vi "workspace.add_to_payload.vi"(8 "error in":errorcluster, 10 "JSON payload in":string, 11 "Nominal Client in":refnum<class "Nominal Client.lvclass">) -> (0 "error out":errorcluster, 1 "JSON payload out":string, 3 "Nominal Client out":refnum<class "Nominal Client.lvclass">)   [LabVIEW 2020, in "Nominal Client.lvclass"]
uses:
  Nominal Client.lvclass
  Nominal Client.lvclass/Nominal Client.ctl
  nominal types/workspace/workspace.lvclass/workspace.ctl
  88650e10-de3e-481c-85db-71cb0fdf4485.vi
  nominal types/workspace/rid.get.vi
  <vilib>/JDP Science/JSONtext/Variant to JSON Text.vi
  <vilib>/JDP Science/JSONtext/Get all Object Items.vi
  <vilib>/JDP Science/JSONtext/Set Multiple Object Items.vi
  <vilib>/JDP Science/JSONtext/LVClass Serializer/JSONtext LVClass Serializer.lvclass
  <vilib>/JDP Science/JSONtext/JSONtext.lvlib
  nominal types/workspace/workspace.lvclass
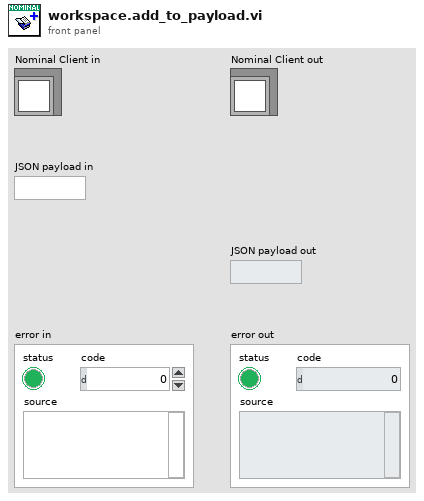
[diagram p1: front panel]
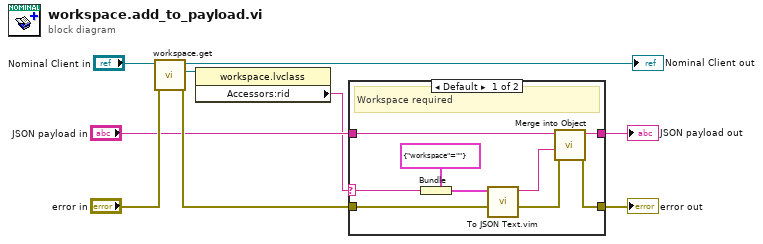
[diagram p0: block diagram]
diagram:
  n1 = call "workspace.get.vi"("error in"="error in", "Nominal Client in"="Nominal Client in") -> ("error out"=w6:errorcluster, "workspace"=w2:refnum<class "workspace.lvclass">, "Nominal Client out"=→"Nominal Client out":refnum<class "Nominal Client.lvclass">)  [unwired: 7 in]
  n2 = property class="workspace.lvclass"(reference=w2) -> ("Accessors:rid"=w1:string)  [unwired: 1 in, 2 out]
  n3 = case shown="Default" w1 {
    selector: w1 -> [w12 _]
    tunnel: [w17 w20] -> w8
    tunnel: "JSON payload in" -> [w18 w20]
    tunnel: [w16 w19] -> w7
    tunnel: w6 -> [w15 w19]
    frame Default {
      # "Workspace required"
      n4 = Bundle(cluster=cluster{"workspace":string} {"workspace"=""}, "workspace"=w12) -> (w10:cluster{"workspace":string})
      n5 = call "To JSON Text.vim"("error in (no error)"=w15, "Anything"=w10) -> ("error out"=w13:errorcluster, "<JSON>"=w14:string)  [unwired: 8 in]
      n6 = call <vilib>:"Merge into Object.vi"("error in (no error)"=w13, "JSON Object to Merge"=w14, "JSON"=w18) -> ("error out"=w16:errorcluster, "<JSON>"=w17:string)  [unwired: 6 in]
    }
    frame "" {
      # "Not using a workspace"
    }
  }
  "JSON payload out" <- w8
  "error out" <- w7
